vi "Auton - Boiler Gear Shoot.vi"(9 "Alliance":T2, 11 "Auton States":T1=enum."Reset Encoders") -> ()   [LabVIEW 2016]
uses:
  Auton - Boiler Gear Shoot States.ctl
  <vilib>/Rock Robotics/WPI/DriverStation/WPI_DriverStationAllianceInfo.ctl
  Robot Values.vi
panel:
  in  "High Speed Output Range":cluster{"output high":dbl, "output low":dbl}={"output high"=0.9, "output low"=-0.9}
  out "Auton State":T1=enum."Shoot"
  in  "Mount Gear SP":dbl=14.0
  in  "Blue - Mount Gear Turn":dbl=58.0 format="%#_13g"
  in  "Red - Mount Gear Turn":dbl=302.0 format="%#_13g"
  in  "Blue - Turn to Boiler":dbl=217.0 format="%#_13g"
  in  "Red - Turn to Boiler SP":dbl=143.0 format="%#_13g"
  in  "Move to Boiler SP":dbl=101.0
  in  "Back Away Gear SP":dbl=3.0
  in  "Red - Face Airship Setpoint":dbl=286.0 format="%#_13g"
  in  "Go to Vision Target SP":dbl=50.0
  in  "Blue - Face Airship Setpoint":dbl=74.0 format="%#_13g"
  in  "Drive Forward SP":dbl=77.0
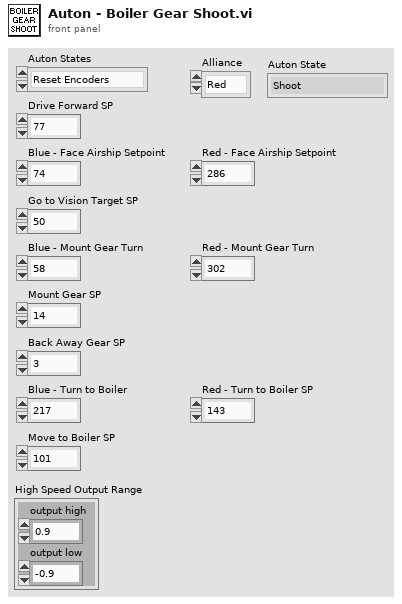
[diagram p1: front panel]
types:
  T1 = typedef "Auton - Boiler Gear Shoot States.ctl" = enum16{"Stop", "Reset Encoders", "Drive Forward", "Face Airship Gyro", "Reset Encoders Again", "Go to Target", "Turn to Mount Gear", "Reset Encoders Mount", "Mount Gear", "Eject Gear", "Back Away from Gear", "Turn to Boiler", "Reset Encoders Boiler", "Move to Boiler", "Shoot", "Back Away from Boiler"}
  T2 = typedef "WPI_DriverStationAllianceInfo.ctl" = enum16{"Red", "Blue", "Invalid"}
  T3 = typedef "Robot Values.ctl" = cluster{"Robot Drive":cluster{"Left Motor Power":dbl, "Right Motor Power":dbl, "Left Encoder Value":dbl, "Right Encoder Value":dbl, "High Gear?":bool, "PTO?":bool}, "Sensors":cluster{"Gyro Angle":u16, "Recalibrate Gyro":bool, "Reset Gyro":bool, "Ultrasonic":dbl}, "Shooter":cluster{"Prep Wheels":bool, "Shoot":bool, "Left Shooter Wheel Speed":dbl, "Wheels Moving":bool, "Shooter Prepped":bool, "Shooter RPS SP":dbl, "Shooting?":bool, "Left Shooter Wheel Power":dbl, "Right Shooter Wheel Power":dbl, "Acquisition Conveyor Power":dbl, "Hopper Beater Bar Power":dbl, "Filtered Left Shooter Speed":dbl, "Acquisition Motor Power":dbl, "Joystick Add":dbl, "D-Pad Add":dbl, "Shooter Use PID?":bool}, "Robot States":cluster{"Drive mode":string, "Alliance":T2, "Position":T4}, "Gear":cluster{"Ejection Active":bool}}
  T4 = typedef "WPI_DriverStationPositionInfo.ctl" = enum16{"1", "2", "3"}
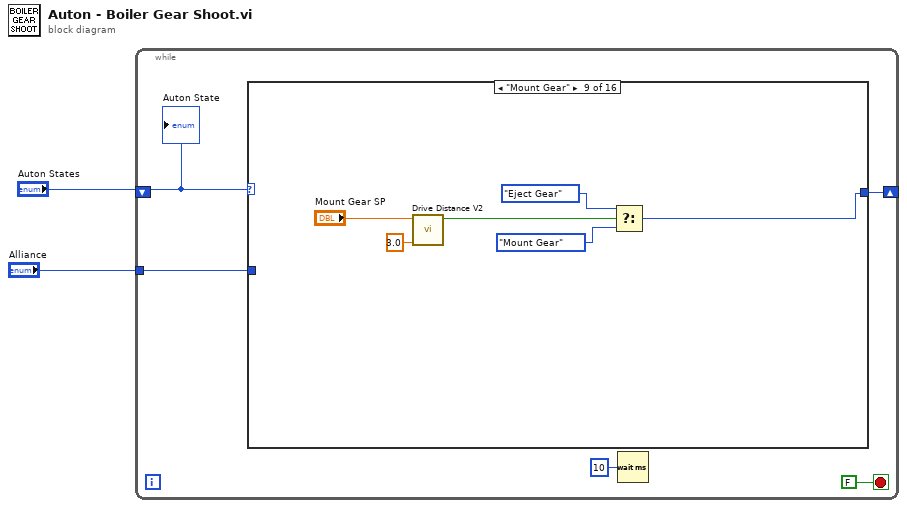
[diagram p0: block diagram]
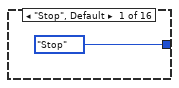
[diagram p2: hidden frame]
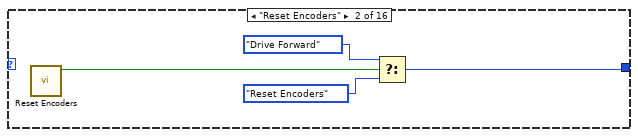
[diagram p3: hidden frame]
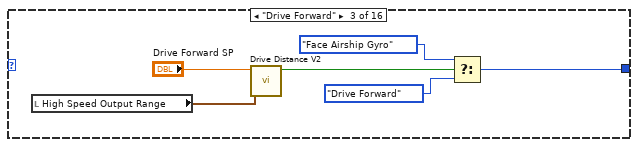
[diagram p4: hidden frame]
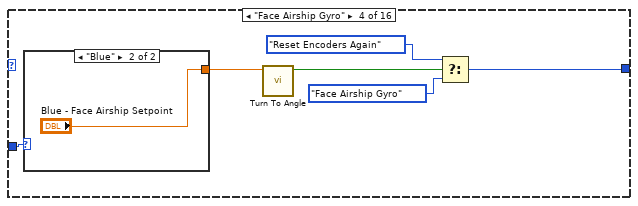
[diagram p5: hidden frame]
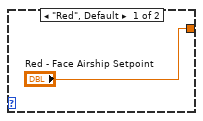
[diagram p6: hidden frame]
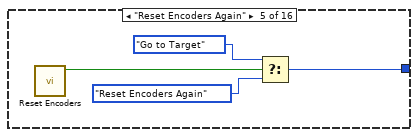
[diagram p7: hidden frame]
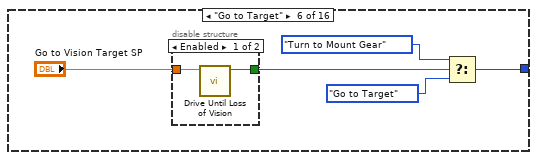
[diagram p8: hidden frame]
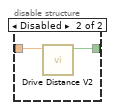
[diagram p9: hidden frame]
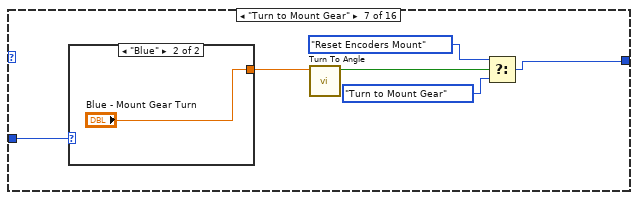
[diagram p10: hidden frame]
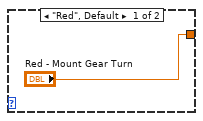
[diagram p11: hidden frame]
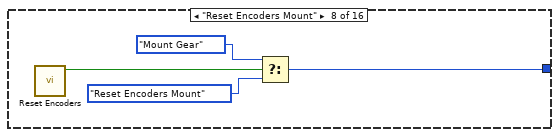
[diagram p12: hidden frame]
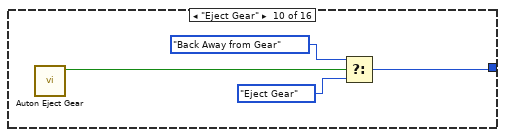
[diagram p13: hidden frame]
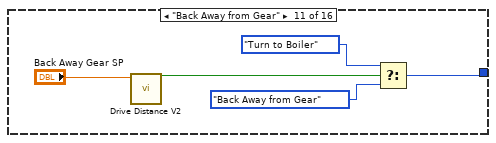
[diagram p14: hidden frame]
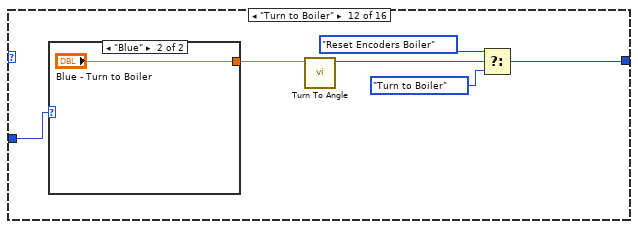
[diagram p15: hidden frame]
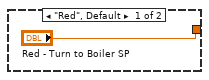
[diagram p16: hidden frame]
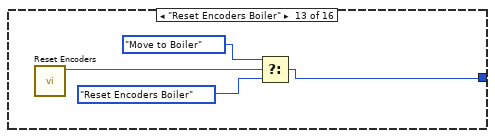
[diagram p17: hidden frame]
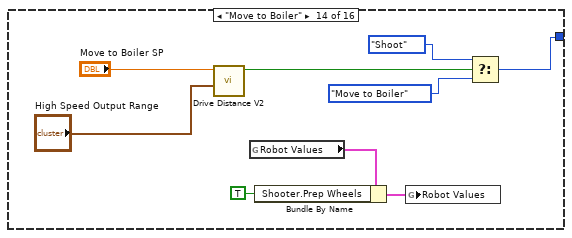
[diagram p18: hidden frame]
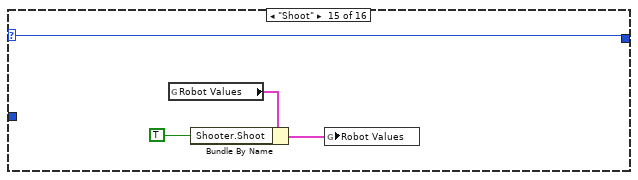
[diagram p19: hidden frame]
diagram:
  n1 = while {
    shift-right: [w6] -> _
    shift-left: "Auton States" -> [w7]
    tunnel: "Alliance" -> [w5]
    stop <- FALSE stop-if-true
    n2 = case shown="\"Mount Gear\"" w7 {
      selector: w7 -> [_ _ _ _ _ _ _ _ _ _ _ _ _ _ w88 _]
      tunnel: [Auton_-_Boiler_Gear_Shoot_States."Stop" ("Auton States") w11 w16 w22 w28 w33 w41 w48 w57 w59 w64 w69 w76 w83 w88 _] -> w6
      tunnel: w5 -> [_ _ _ w19 _ _ w40 _ _ _ _ w68 _ _ _ _]
      frame "Stop", Default {
      }
      frame "Reset Encoders" {
        n3 = call "Reset Encoders.vi"() -> ("Done?"=w12:bool)  [unwired: 11 in]
        n4 = Select(t=Auton_-_Boiler_Gear_Shoot_States."Drive Forward" ("Auton States"), s=w12, f=Auton_-_Boiler_Gear_Shoot_States."Reset Encoders" ("Auton States")) -> (s? t:f=w11:T1)
      }
      frame "Drive Forward" {
        n5 = local read "High Speed Output Range"() -> (w13:cluster{"output high":dbl, "output low":dbl})
        n6 = call "Drive Distance V2.vi"("output range"=w13, "Distance Set Point"="Drive Forward SP") -> ("Done?"=w15:bool)  [unwired: 9 in]
        n7 = Select(t=Auton_-_Boiler_Gear_Shoot_States."Face Airship Gyro" ("Auton States"), s=w15, f=Auton_-_Boiler_Gear_Shoot_States."Drive Forward" ("Auton States")) -> (s? t:f=w16:T1)
      }
      frame "Face Airship Gyro" {
        n8 = case shown="\"Blue\"" w19 {
          tunnel: ["Red - Face Airship Setpoint" "Blue - Face Airship Setpoint"] -> w20
          frame "Red", Default {
          }
          frame "Blue" {
          }
        }
        n9 = call "Turn To Angle.vi"("Setpoint"=w20) -> ("Done?"=w21:bool)  [unwired: 10 in]
        n10 = Select(t=Auton_-_Boiler_Gear_Shoot_States."Reset Encoders Again" ("Auton States"), s=w21, f=Auton_-_Boiler_Gear_Shoot_States."Face Airship Gyro" ("Auton States")) -> (s? t:f=w22:T1)
      }
      frame "Reset Encoders Again" {
        n11 = call "Reset Encoders.vi"() -> ("Done?"=w27:bool)  [unwired: 11 in]
        n12 = Select(t=Auton_-_Boiler_Gear_Shoot_States."Go to Target" ("Auton States"), s=w27, f=Auton_-_Boiler_Gear_Shoot_States."Reset Encoders Again" ("Auton States")) -> (s? t:f=w28:T1)
      }
      frame "Go to Target" {
        n13 = disable-structure shown="Enabled" {
          disable-tunnel: [w37 w38] -> w32
          disable-tunnel: "Go to Vision Target SP" -> [w36 w39]
          frame Enabled {
            n14 = call "Drive Until Loss of Vision.vi"("Distance Setpoint"=w36) -> ("ready to approach"=w37:bool)  [unwired: 10 in]
          }
          frame Disabled {
            n15 = call "Drive Distance V2.vi"("Distance Set Point"=w39) -> ("Done?"=w38:bool)  [unwired: 10 in]
          }
        }
        n16 = Select(t=Auton_-_Boiler_Gear_Shoot_States."Turn to Mount Gear" ("Auton States"), s=w32, f=Auton_-_Boiler_Gear_Shoot_States."Go to Target" ("Auton States")) -> (s? t:f=w33:T1)
      }
      frame "Turn to Mount Gear" {
        n17 = case shown="\"Blue\"" w40 {
          tunnel: ["Red - Mount Gear Turn" "Blue - Mount Gear Turn"] -> w42
          frame "Red", Default {
          }
          frame "Blue" {
          }
        }
        n18 = call "Turn To Angle.vi"("Setpoint"=w42) -> ("Done?"=w43:bool)  [unwired: 10 in]
        n19 = Select(t=Auton_-_Boiler_Gear_Shoot_States."Reset Encoders Mount" ("Auton States"), s=w43, f=Auton_-_Boiler_Gear_Shoot_States."Turn to Mount Gear" ("Auton States")) -> (s? t:f=w41:T1)
      }
      frame "Reset Encoders Mount" {
        n20 = call "Reset Encoders.vi"() -> ("Done?"=w49:bool)  [unwired: 11 in]
        n21 = Select(t=Auton_-_Boiler_Gear_Shoot_States."Mount Gear" ("Auton States"), s=w49, f=Auton_-_Boiler_Gear_Shoot_States."Reset Encoders Mount" ("Auton States")) -> (s? t:f=w48:T1)
      }
      frame "Mount Gear" {
        n22 = call "Drive Distance V2.vi"("Tolerance"=3.0, "Distance Set Point"="Mount Gear SP") -> ("Done?"=w54:bool)  [unwired: 9 in]
        n23 = Select(t=Auton_-_Boiler_Gear_Shoot_States."Eject Gear" ("Auton States"), s=w54, f=Auton_-_Boiler_Gear_Shoot_States."Mount Gear" ("Auton States")) -> (s? t:f=w57:T1)
      }
      frame "Eject Gear" {
        n24 = call "Auton Eject Gear.vi"() -> ("Done?"=w58:bool)  [unwired: 11 in]
        n25 = Select(t=Auton_-_Boiler_Gear_Shoot_States."Back Away from Gear" ("Auton States"), s=w58, f=Auton_-_Boiler_Gear_Shoot_States."Eject Gear" ("Auton States")) -> (s? t:f=w59:T1)
      }
      frame "Back Away from Gear" {
        n26 = call "Drive Distance V2.vi"("Distance Set Point"="Back Away Gear SP") -> ("Done?"=w63:bool)  [unwired: 10 in]
        n27 = Select(t=Auton_-_Boiler_Gear_Shoot_States."Turn to Boiler" ("Auton States"), s=w63, f=Auton_-_Boiler_Gear_Shoot_States."Back Away from Gear" ("Auton States")) -> (s? t:f=w64:T1)
      }
      frame "Turn to Boiler" {
        n28 = case shown="\"Blue\"" w68 {
          tunnel: ["Red - Turn to Boiler SP" "Blue - Turn to Boiler"] -> w70
          frame "Red", Default {
          }
          frame "Blue" {
          }
        }
        n29 = call "Turn To Angle.vi"("Setpoint"=w70) -> ("Done?"=w71:bool)  [unwired: 10 in]
        n30 = Select(t=Auton_-_Boiler_Gear_Shoot_States."Reset Encoders Boiler" ("Auton States"), s=w71, f=Auton_-_Boiler_Gear_Shoot_States."Turn to Boiler" ("Auton States")) -> (s? t:f=w69:T1)
      }
      frame "Reset Encoders Boiler" {
        n31 = call "Reset Encoders.vi"() -> ("Done?"=w77:bool)  [unwired: 11 in]
        n32 = Select(t=Auton_-_Boiler_Gear_Shoot_States."Move to Boiler" ("Auton States"), s=w77, f=Auton_-_Boiler_Gear_Shoot_States."Reset Encoders Boiler" ("Auton States")) -> (s? t:f=w76:T1)
      }
      frame "Move to Boiler" {
        n33 = call "Drive Distance V2.vi"("output range"="High Speed Output Range", "Distance Set Point"="Move to Boiler SP") -> ("Done?"=w86:bool)  [unwired: 9 in]
        n34 = global read "Robot Values.vi" "Robot Values"() -> (w82:T3)
        n35 = Bundle By Name(cluster=w82, "Shooter.Prep Wheels"=TRUE) -> (w81:T3)
        n36 = global write "Robot Values.vi" "Robot Values"(w81) -> ()
        n37 = Select(t=Auton_-_Boiler_Gear_Shoot_States."Shoot" ("Auton States"), s=w86, f=Auton_-_Boiler_Gear_Shoot_States."Move to Boiler" ("Auton States")) -> (s? t:f=w83:T1)
      }
      frame "Shoot" {
        n38 = global read "Robot Values.vi" "Robot Values"() -> (w91:T3)
        n39 = Bundle By Name(cluster=w91, "Shooter.Shoot"=TRUE ("Shooter.Prep Wheels")) -> (w90:T3)
        n40 = global write "Robot Values.vi" "Robot Values"(w90) -> ()
      }
      frame "Back Away from Boiler" {
      }
    }
    n41 = Wait (ms)(milliseconds to wait=u32 10) -> ()  [unwired: 1 out]
    "Auton State" <- w7
  }
